vi "MJG_StageRefFollower_v1.vi"(8 "error in":errorcluster, 9 "Stage PID Cluster":T1={"Stage Z PID"={"Kp"=0.0003, "Kd"=0.01, "Ki"=0.0}, "Stage Y PID"={"Kp"=0.0003, "Kd"=0.01, "Ki"=0.0}, "Stage X PID"={"Kp"=0.0003, "Kd"=0.01, "Ki"=0.0}}, 10 "Stage cmd Posit [mm]":dbl[](array[numeric])=[6.0, 6.0, 6.0], 11 "Refnum In":refnum<k20>) -> (0 "error out":errorcluster, 2 "Stage out Posit [mm]":dbl[](array[numeric])=[12.0, 0.0, 0.0], 3 "Refnum out":refnum<k20>)   [LabVIEW 2016]
uses:
  <vilib>/Utility/error.llb/Error Cluster From Error Code.vi
  <vilib>/rvi/errors/niLvFpgaAdjustHostInterfaceError.vi
  Subsystems/GLOBALVARS.vi
  <vilib>/rvi/interface/nirviReadWriteControl/nirviReadWriteControl.xnode
  FPGA Bitfiles/IRISSTeleoperati_FPGATarget_IRISSFPGAIOv2_C6m-myIOTk0.lvbitx
  FPGA/IRISS_FPGA_IO_v2.vi
  NiFpgaLv.dll
panel:
  # ">>>"
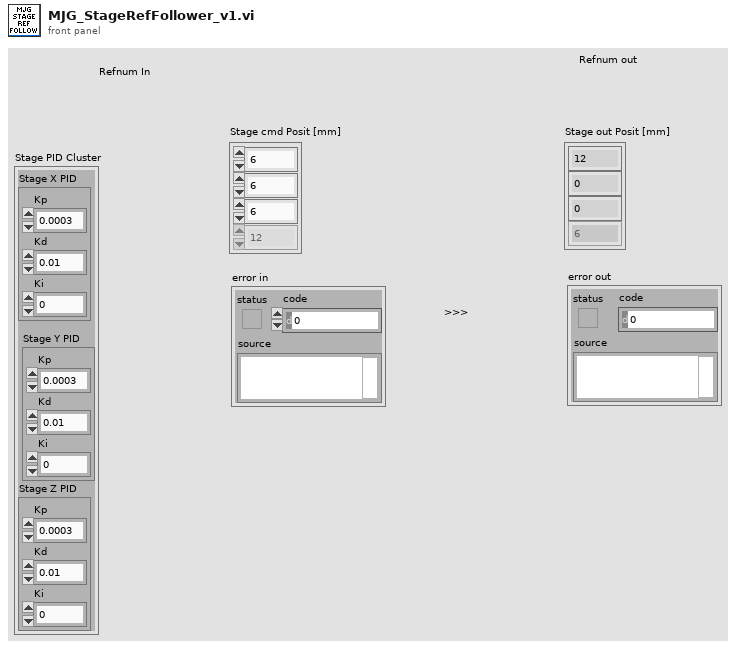
[diagram p1: front panel]
types:
  T1 = cluster{"Stage Z PID":cluster{"Kp":dbl, "Kd":dbl, "Ki":dbl}, "Stage Y PID":cluster{"Kp":dbl, "Kd":dbl, "Ki":dbl}, "Stage X PID":cluster{"Kp":dbl, "Kd":dbl, "Ki":dbl}}
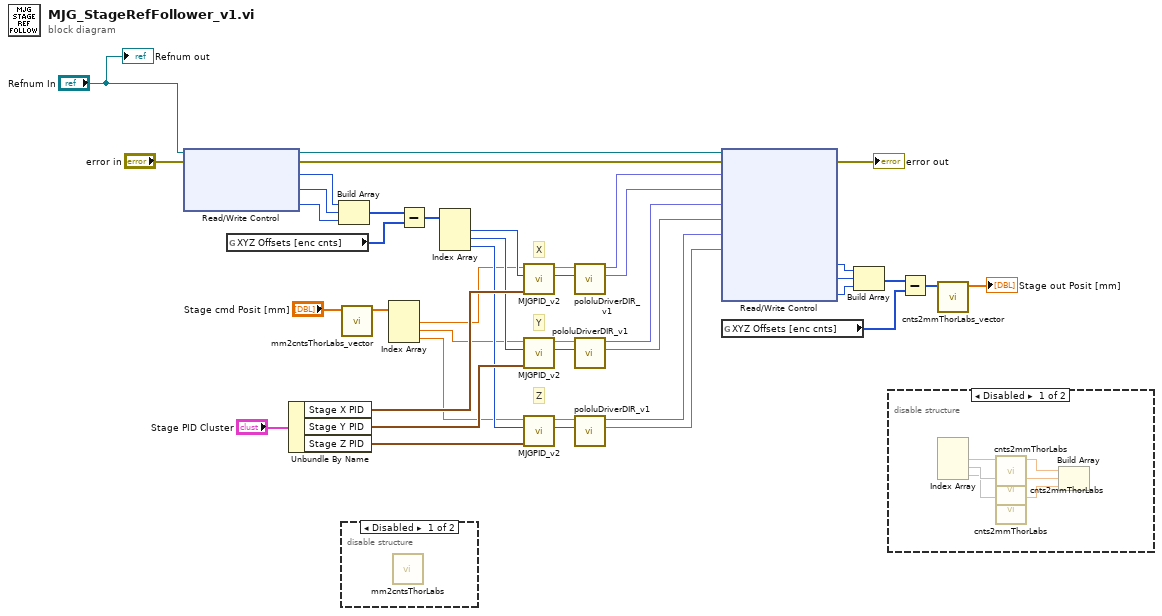
[diagram p0: block diagram]
diagram:
  # "X"
  # "Y"
  # "Z"
  n1 = xnode "Read/Write Control"("FPGA VI Reference In"="Refnum In", "error in"="error in") -> ("FPGA VI Reference Out"=w33:refnum<k20>, "error out"=w32:errorcluster, "X Stage Enc Count"=w18:i32, "Y Stage Enc Count"=w16:i32, "Z Stage Enc Count"=w14:i32)
  n2 = global read "GLOBALVARS.vi" "XYZ Offsets [enc cnts]"() -> (w20:i32[])
  n3 = Unbundle By Name("Stage PID Cluster") -> ("Stage X PID"=w24:cluster{"Kp":dbl, "Kd":dbl, "Ki":dbl}, "Stage Y PID"=w23:cluster{"Kp":dbl, "Kd":dbl, "Ki":dbl}, "Stage Z PID"=w22:cluster{"Kp":dbl, "Kd":dbl, "Ki":dbl})
  n4 = Build Array(w18, w16, w14) -> (w21:i32[])
  n5 = call "mm2cntsThorLabs_vector.vi"("XYZ cmd [mm]"="Stage cmd Posit [mm]") -> ("XYZ cmd [enc cnts]"=w1:dbl[])  [unwired: 10 in]
  n6 = disable-structure shown="Disabled" {
    frame Disabled {
      n7 = call "mm2cntsThorLabs.vi"() -> ()  [unwired: 11 in, 1 out]
    }
    frame Enabled {
    }
  }
  n8 = Index Array(array=w1) -> (element #1=w5:dbl, element #2=w4:dbl, element #3=w3:dbl)  [unwired: 3 in]
  n9 = Subtract(x=w21, y=w20) -> (x-y=w19:i32[])
  n10 = Index Array(array=w19) -> (element #1=w17:i32, element #2=w15:i32, element #3=w13:i32)  [unwired: 3 in]
  n11 = call "MJGPID_v2.vi"("PID Gains"=w24, "Encoder Position"=w17, "Reference"=w5) -> ("Direction"=w30:bool, "Duty Cycle"=w31:dbl)  [unwired: 7 in]
  n12 = call "MJGPID_v2.vi"("PID Gains"=w23, "Encoder Position"=w15, "Reference"=w4) -> ("Direction"=w28:bool, "Duty Cycle"=w29:dbl)  [unwired: 7 in]
  n13 = call "MJGPID_v2.vi"("PID Gains"=w22, "Encoder Position"=w13, "Reference"=w3) -> ("Direction"=w26:bool, "Duty Cycle"=w27:dbl)  [unwired: 7 in]
  n14 = call "pololuDriverDIR_v1.vi"("Direction"=w30, "Duty Cycle"=w31) -> ("PWM 2 Out"=w40:fxp<+,32,0>, "PWM 1 Out"=w41:fxp<+,32,0>)  [unwired: 8 in]
  n15 = call "pololuDriverDIR_v1.vi"("Direction"=w28, "Duty Cycle"=w29) -> ("PWM 2 Out"=w39:fxp<+,32,0>, "PWM 1 Out"=w38:fxp<+,32,0>)  [unwired: 8 in]
  n16 = call "pololuDriverDIR_v1.vi"("Direction"=w26, "Duty Cycle"=w27) -> ("PWM 2 Out"=w36:fxp<+,32,0>, "PWM 1 Out"=w37:fxp<+,32,0>)  [unwired: 8 in]
  n17 = xnode "Read/Write Control"("FPGA VI Reference In"=w33, "error in"=w32, "X PWM 1"=w41, "X PWM 2"=w40, "Y PWM 1"=w38, "Y PWM 2"=w39, "Z PWM 1"=w37, "Z PWM 2"=w36) -> ("error out"=→"error out":errorcluster, "X Stage Enc Count"=w12:i32, "Y Stage Enc Count"=w11:i32, "Z Stage Enc Count"=w10:i32)  [unwired: 1 out]
  n18 = global read "GLOBALVARS.vi" "XYZ Offsets [enc cnts]"() -> (w8:i32[])
  n19 = Build Array(w12, w11, w10) -> (w9:i32[])
  n20 = disable-structure shown="Disabled" {
    frame Disabled {
      n21 = Index Array() -> (element #1=w45, element #2=w44, element #3=w43)  [unwired: 4 in]
      n22 = call "cnts2mmThorLabs.vi"("XYX cmd [enc cnts]"=w45) -> ("XYZ cmd [mm]"=w48:dbl)  [unwired: 10 in]
      n23 = call "cnts2mmThorLabs.vi"("XYX cmd [enc cnts]"=w44) -> ("XYZ cmd [mm]"=w47:dbl)  [unwired: 10 in]
      n24 = call "cnts2mmThorLabs.vi"("XYX cmd [enc cnts]"=w43) -> ("XYZ cmd [mm]"=w46:dbl)  [unwired: 10 in]
      n25 = Build Array(w48, w47, w46) -> ()  [unwired: 1 out]
    }
    frame Enabled {
    }
  }
  n26 = Subtract(x=w9, y=w8) -> (x-y=w7:i32[])
  n27 = call "cnts2mmThorLabs_vector.vi"("XYZ cmd [end cnts]"=w7) -> ("XYZ cmd [mm]"=→"Stage out Posit [mm]":dbl[])  [unwired: 10 in]
  "Refnum out" <- "Refnum In"
